vi "GetPresetsPresent.vi"(8 "error in (no error)":errorcluster, 11 "Gviewer in":refnum<class "Gviewer.lvclass">) -> (0 "error out":errorcluster, 1 "PresentsInMenu":T1[](array[typedef]), 3 "Gviewer out":refnum<class "Gviewer.lvclass">)   [LabVIEW 2020, in "Sgraph_lib_V1.lvlib" / "Gviewer.lvclass"]
doc: "Delivers the number of presets present for the preset menu"
uses:
  Gviewer.lvclass
  menu/MenuItem.ctl
  Gviewer.lvclass/Gviewer.ctl
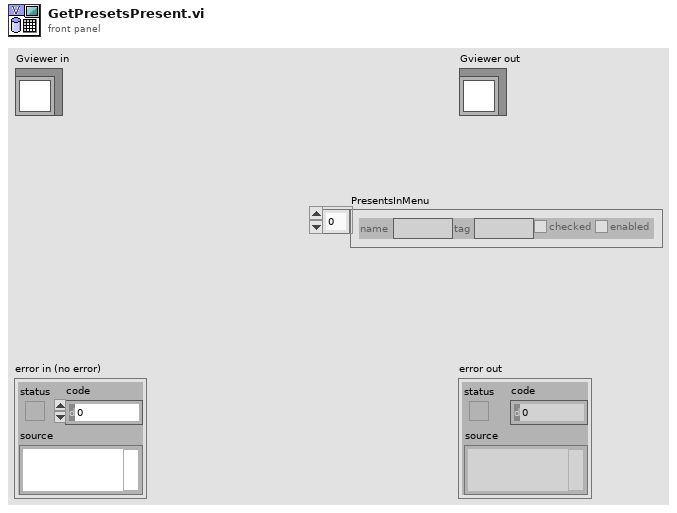
[diagram p1: front panel]
types:
  T1 = typedef "MenuItem.ctl" = cluster{"name":string, "tag":string, "checked":bool, "enabled":bool}
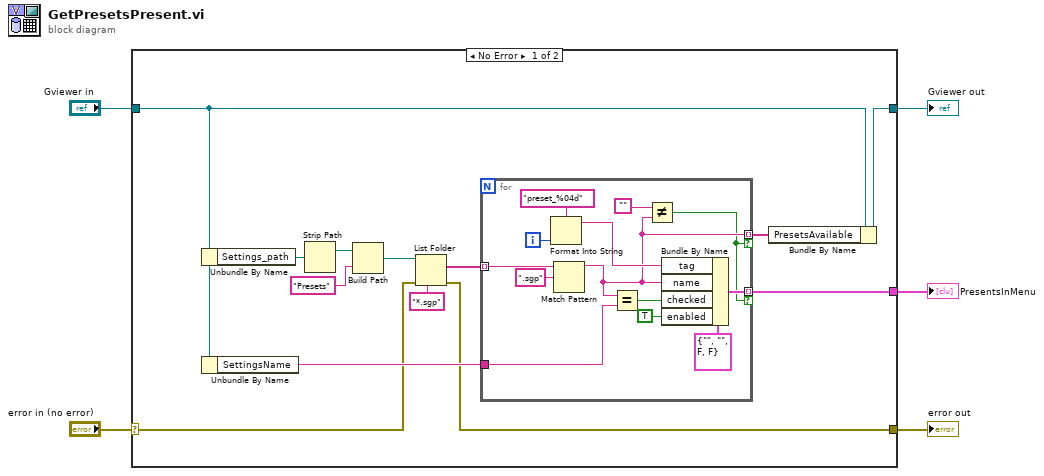
[diagram p0: block diagram]
diagram:
  n1 = case shown="No Error" "error in (no error)" {
    selector: "error in (no error)" -> [w13 w33]
    tunnel: [w12 w33] -> w4
    tunnel: [w10 w32] -> w2
    tunnel: "Gviewer in" -> [w9 w32]
    tunnel: [w11 _] -> w1
    frame No Error {
      n2 = Unbundle By Name(w9) -> ("Settings_path"=w18:path)
      n3 = Unbundle By Name(w9) -> ("SettingsName"=w14:string)
      n4 = Strip Path(path=w18) -> (stripped path=w17:path)  [unwired: 1 out]
      n5 = Build Path(base path=w17, name or relative path="Presets") -> (appended path=w8:path)
      n6 = List Folder(path=w8, pattern="*.sgp", error in=w13) -> (filenames=w7:string[], error out=w12:errorcluster)  [unwired: 1 in, 2 out]
      n7 = for {
        tunnel: w7 -> [w22] mode=indexing
        tunnel: w14 -> [w28]
        tunnel: [w26] -> w11 mode=indexing if=w19
        tunnel: [w21] -> w6 mode=indexing if=w19
        i -> [w24]
        n8 = Format Into String(format string="preset_%04d", w24) -> (resulting string=w23:string)  [unwired: 2 in, 1 out]
        n9 = Match Pattern(string=w22, regular expression=".sgp" ("pattern")) -> (before substring=w21:string)  [unwired: 1 in, 3 out]
        n10 = Equal?(x=w21, y=w28) -> (x = y?=w27:bool)
        n11 = Not Equal?(x="", y=w21) -> (x != y?=w19:bool)
        n12 = Bundle By Name(cluster=T1 {"name"="", "tag"="", "checked"=FALSE, "enabled"=FALSE} ("menu-item"), "tag"=w23, "name"=w21, "checked"=w27, "enabled"=TRUE) -> (w26:T1)
      }
      n13 = Bundle By Name(cluster=w9, "PresetsAvailable"=w6) -> (w10:refnum<class "Gviewer.lvclass">)
    }
    frame Error {
    }
  }
  "error out" <- w4
  "Gviewer out" <- w2
  "PresentsInMenu" <- w1
